vi "update全局.vi"() -> ()   [LabVIEW 2016, in "自动更新.lvlib"]
panel:
  out "软件版本":string
  in  "updateconfiguration":cluster{"IP地址":string, "端口号":i32}={"IP地址"="27.154.58.30", "端口号"=11234}
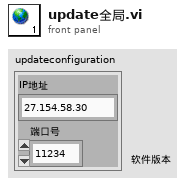
[diagram p1: front panel]
diagram:
